vi "Calculate Total Tardiness for Brucker Instance.vi"() -> ()   [LabVIEW 2013]
uses:
  <vilib>/Heliosphere Research LLC/Advanced Plotting Toolkit/typedefs/PlotColor.ctl
  <vilib>/Heliosphere Research LLC/Advanced Plotting Toolkit/api_figure/TicksProperties.ctl
  <vilib>/Heliosphere Research LLC/Advanced Plotting Toolkit/properties/Text.ctl
  <vilib>/Heliosphere Research LLC/Advanced Plotting Toolkit/properties/Text_FontSize.ctl
  <vilib>/Heliosphere Research LLC/Advanced Plotting Toolkit/properties/Text_FontStyle.ctl
  <vilib>/Heliosphere Research LLC/Advanced Plotting Toolkit/api_annotations/ShapeProperties.ctl
  <vilib>/Heliosphere Research LLC/Advanced Plotting Toolkit/properties/Line.ctl
  <vilib>/Heliosphere Research LLC/Advanced Plotting Toolkit/properties/Line_Style.ctl
  <vilib>/Heliosphere Research LLC/Advanced Plotting Toolkit/properties/Display.ctl
  <vilib>/Heliosphere Research LLC/Advanced Plotting Toolkit/api_annotations/TextProperties.ctl
  Classes/Scheduler_Class/Check Other Machines for Schedule Time.vi
  Classes/Scheduler_Class/Schedule Job.vi
  Classes/Scheduler_Class/Find Gaps on Particular Machine.vi
  Classes/Scheduler_Class/Increment Number of Jobs on Machine.vi
  Classes/Scheduler_Class/Operation to Machine Job Tuple.vi
  Classes/Scheduler_Class/Find Job On Other Machines.vi
  Classes/Scheduler.lvclass
  <vilib>/Heliosphere Research LLC/Advanced Plotting Toolkit/Advanced Plotting Toolkit.lvlib
panel:
  out "Picture":picture
  out "sum":i32
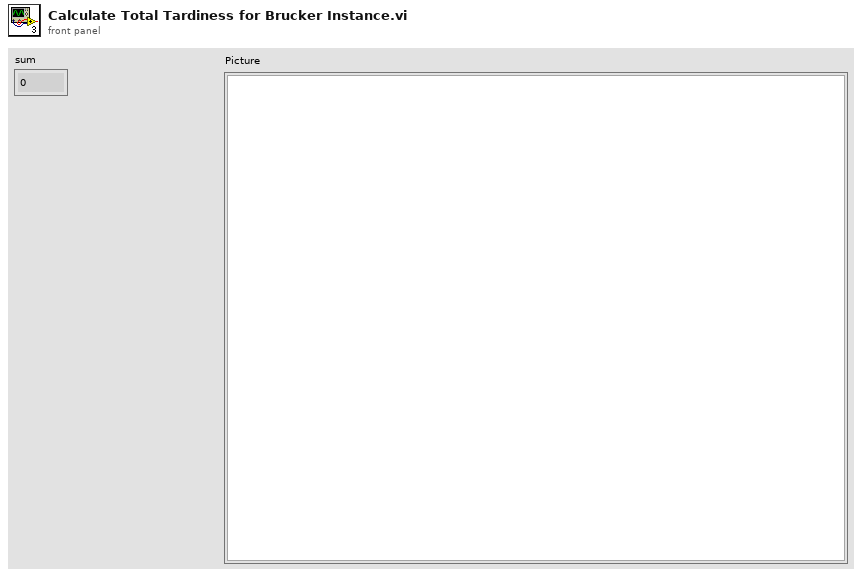
[diagram p1: front panel]
types:
  T1 = typedef "GanntChart_Element.ctl" = cluster{"Operation Number":i32, "Job Number":i32, "Start Time":i32, "Procesing Time":u16, "End Time":i32}
  T2 = typedef "Advanced Plotting Toolkit.lvlib/TicksProperties.ctl" = cluster{"Text":T3}
  T3 = typedef "Advanced Plotting Toolkit.lvlib/Text.ctl" = cluster{"Color":T4, "Background Color":T4, "Font Size (points)":T5, "Font Style":T6, "Rotation Angle":dbl}
  T4 = typedef "Advanced Plotting Toolkit.lvlib/PlotColor.ctl" = u32
  T5 = typedef "Advanced Plotting Toolkit.lvlib/Text_FontSize.ctl" = i32
  T6 = typedef "Advanced Plotting Toolkit.lvlib/Text_FontStyle.ctl" = enum16{"Automatic", "Normal", "Italic", "Bold"}
  T7 = typedef "Advanced Plotting Toolkit.lvlib/TextProperties.ctl" = cluster{"Text":T3, "Display":T8}
  T8 = typedef "Advanced Plotting Toolkit.lvlib/Display.ctl" = cluster{"Alpha":dbl, "Z Order":dbl}
  T9 = typedef "Advanced Plotting Toolkit.lvlib/ShapeProperties.ctl" = cluster{"Color":T4, "Line":T10, "Display":T8}
  T10 = typedef "Advanced Plotting Toolkit.lvlib/Line.ctl" = cluster{"Style":T11, "Color":T4, "Width":sgl}
  T11 = typedef "Advanced Plotting Toolkit.lvlib/Line_Style.ctl" = enum16{"Automatic", "Solid", "Dashed", "Dotted", "Dash-dot", "Invisible"}
  T12 = typedef "Advanced Plotting Toolkit.lvlib/PlotID.ctl" = i32
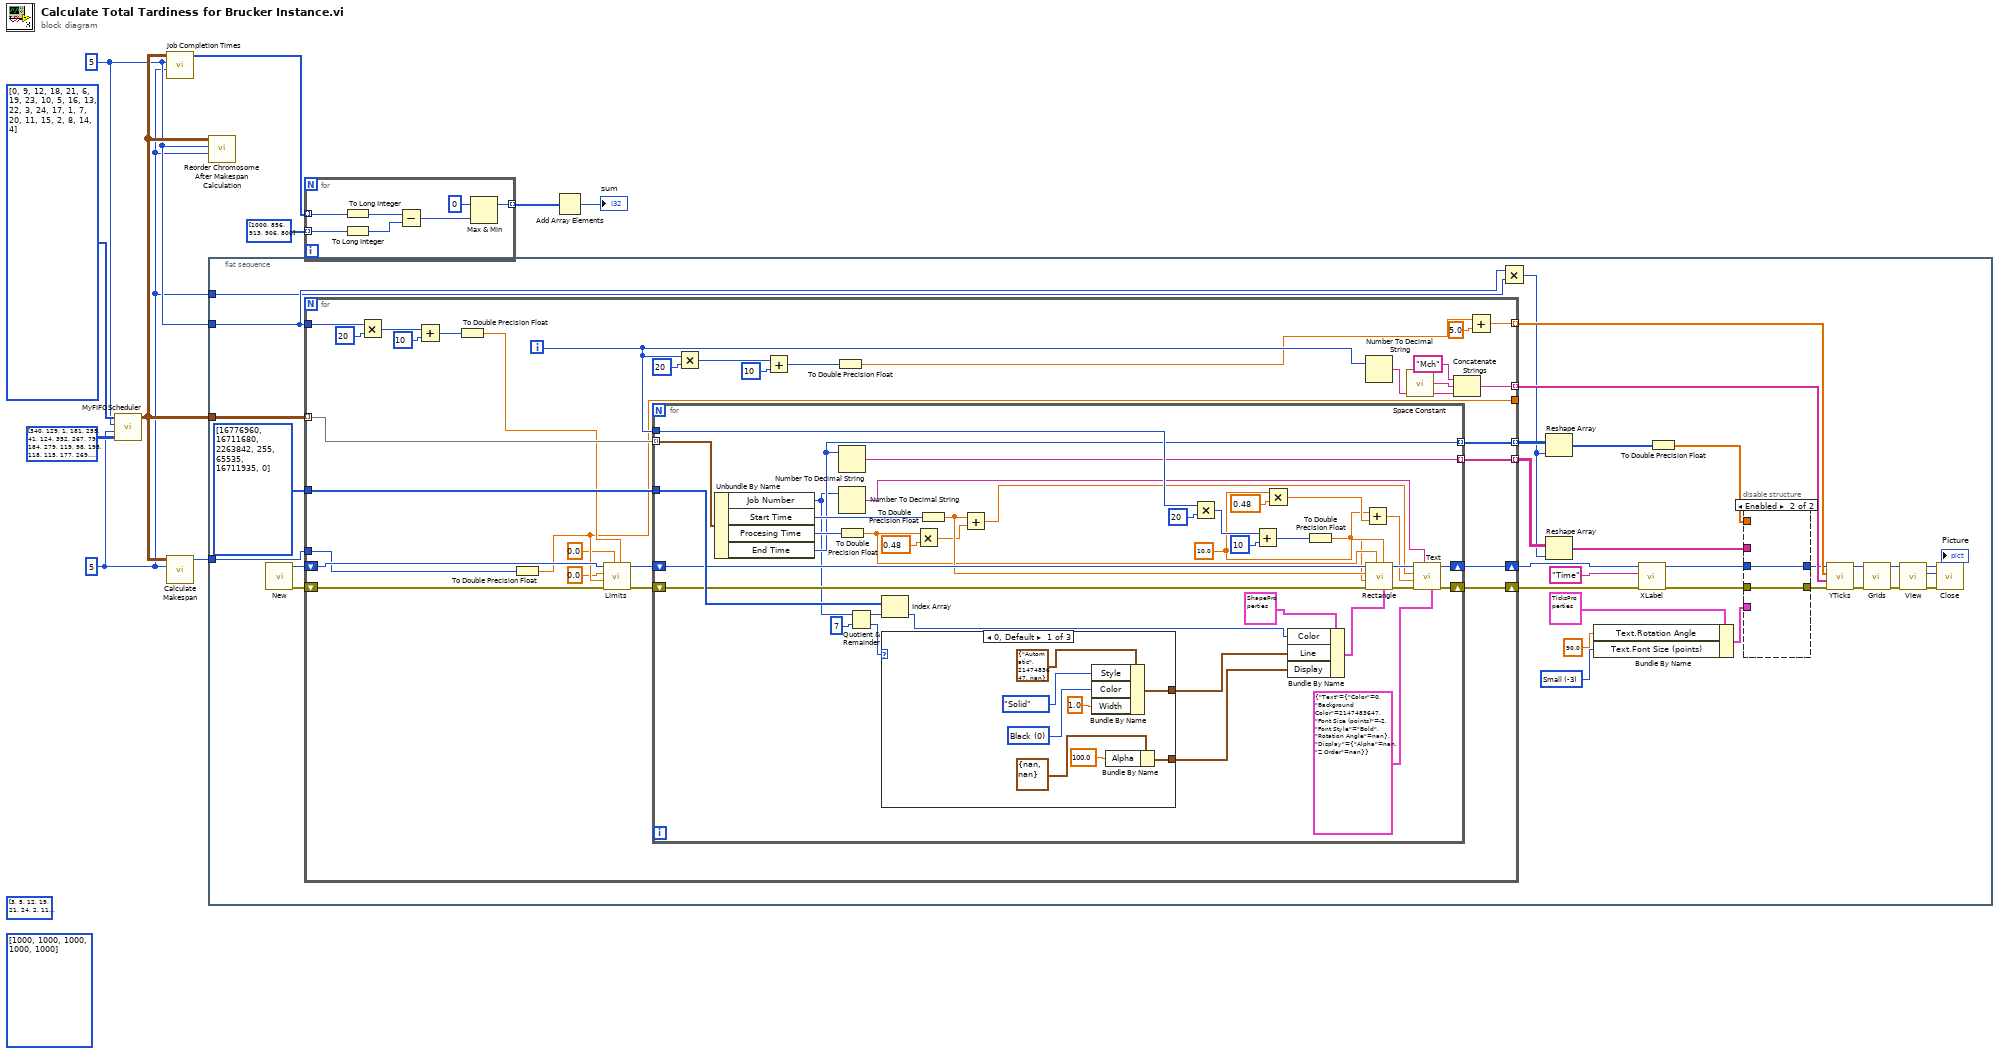
[diagram p0: block diagram]
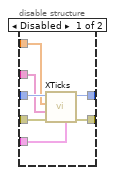
[diagram p2: hidden frame]
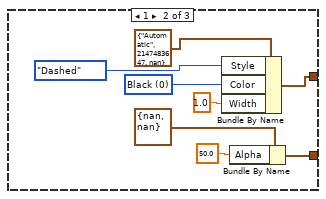
[diagram p3: hidden frame]
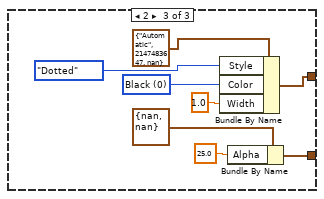
[diagram p4: hidden frame]
diagram:
  (unwired) u16[] [3, 5, 12, 19, 21, 24, 2, 11, 8, 15, 9, 23, 0, 17, 18, 22, 6, 14, 7, 1, 20, 16, 4, 13, 10] ("Schedule")
  (unwired) i32[] [1000, 1000, 1000, 1000, 1000]
  w1 = 5 ("Number of Jobs")
  w2 = 5 ("Number of Machines")
  n1 = call "MyFIFOScheduler.vi"("Processing Times (Rows Mach.Cols Jobs)"=u16[][] [[340, 129, 1, 181, 259], [41, 124, 352, 267, 79], [184, 279, 119, 98, 195], [118, 115, 177, 269, 148], [317, 209, 264, 91, 119]] ("Processing Times"), "Number of Jobs"=w1, "Number of Machines"=w2, "Schedule"=u16[] [0, 9, 12, 18, 21, 6, 19, 23, 10, 5, 16, 13, 22, 3, 24, 17, 1, 7, 20, 11, 15, 2, 8, 14, 4]) -> ("Gannt Chart Out"=w4:T1[][])  [unwired: 6 in, 1 out]
  n2 = call "Job Completion Times.vi"("Number Of Machines"=w1, "Number Of Jobs"=w2, "Gannt Chart In"=w4) -> ("Job Completion Times"=w8:u16[])  [unwired: 8 in]
  n3 = call "Calculate Makespan.vi"("Number of Jobs"=w1, "Gannt Chart In"=w4) -> ("Makespan"=w3:i32)  [unwired: 9 in]
  n4 = call "Reorder Chromosome  After Makespan Calculation.vi"("Number Of  Jobs"=w1, "Number Of Machines"=w2, "Gannt Chart In"=w4) -> ()  [unwired: 8 in, 1 out]
  n5 = flat-sequence {
    tunnel: w4 -> [w16]
    tunnel: w3 -> [w15]
    tunnel: w2 -> [w14]
    tunnel: w1 -> [w13]
    frame #0 {
      w20 = T5 -3 items=["Automatic"=0, "XX-Small"=-1, "X-Small"=-2, "Small"=-3, "Medium"=-4, "Large"=-5, "X-Large"=-6, "XX-Large"=-7] ("Text.Font Size (points)")
      w41 = T4[] [16776960, 16711680, 2263842, 255, 65535, 16711935, 0] items=["Automatic"=2147483647, "Black"=0, "White"=16777215, "Red"=16711680, "Green"=2263842, "Blue"=255, "Cyan"=65535, "Magenta"=16711935, "Yellow"=16776960]
      n6 = call <vilib>:"New.vi"() -> ("error out"=w42:errorcluster, "Plot ID"=w43:T12)  [unwired: 10 in]
      n7 = for {
        shift-right: [w84] -> w39
        shift-left: w42 -> [w80]
        shift-right: [w83] -> w40
        shift-left: w43 -> [w78]
        tunnel: w16 -> [w82] mode=indexing
        tunnel: w41 -> [w81]
        tunnel: [w70] -> w33 mode=indexing
        tunnel: [w60] -> w32 mode=indexing
        tunnel: [w59] -> w19 mode=indexing
        tunnel: [w58] -> w27 mode=indexing
        tunnel: [w57] -> _
        tunnel: w14 -> [w56]
        tunnel: w15 -> [w55]
        i -> [w63]
        n8 = Multiply(x=w56, y=20) -> (x*y=w76:i32)
        n9 = Add(x=w76, y=10) -> (x+y=w74:i32)
        n10 = To Double Precision Float(number=w74) -> (double precision float=w68:dbl)
        n11 = To Double Precision Float(number=w55) -> (double precision float=w57:dbl)
        n12 = call <vilib>:"Limits.vi"("Y Max"=w68, "Y Min"=0.0, "error in (no error)"=w80, "X Max"=w57, "X Min"=0.0, "Plot ID"=w78) -> ("error out"=w79:errorcluster, "Plot ID Out"=w73:T12)  [unwired: 4 in]
        n13 = for {
          shift-right: [w98] -> w84
          shift-left: w79 -> [w120]
          shift-right: [w100] -> w83
          shift-left: w73 -> [w119]
          tunnel: w82 -> [w122] mode=indexing
          tunnel: w81 -> [w121]
          tunnel: w63 -> [w109]
          tunnel: [w103] -> w59 mode=indexing
          tunnel: [w102] -> w58 mode=indexing
          w90 = 10.0 ("Height")
          n14 = Unbundle By Name(w122) -> ("Job Number"=w87:i32, "Start Time"=w114:i32, "Procesing Time"=w115:u16, "End Time"=w103:i32)
          n15 = Number To Decimal String(number=w103) -> (decimal integer string=w102:string)  [unwired: 1 in]
          n16 = Number To Decimal String(number=w87) -> (decimal integer string=w86:string)  [unwired: 1 in]
          n17 = To Double Precision Float(number=w115) -> (double precision float=w96:dbl)
          n18 = Quotient & Remainder(x=w87, y=7) -> (x-y*floor(x/y)=w106:i32, floor(x/y)=w105:i32)
          n19 = Index Array(array=w121, index=w106) -> (element=w116:T4)
          n20 = case shown="0, Default" w105 {
            tunnel: [w126 w134 w142] -> w108
            tunnel: [w123 w131 w139] -> w104
            frame 0, Default {
              w128 = T4 0 items=["Automatic"=2147483647, "Black"=0, "White"=16777215, "Red"=16711680, "Green"=2263842, "Blue"=255, "Cyan"=65535, "Magenta"=16711935, "Yellow"=16776960] ("Color")
              n21 = Bundle By Name(cluster=T10 {"Style"=enum."Automatic", "Color"=2147483647, "Width"=nan} ("Line"), "Style"=Line_Style."Solid", "Color"=w128, "Width"=sgl 1.0) -> (w126:T10)
              n22 = Bundle By Name(cluster=T8 {"Alpha"=nan, "Z Order"=nan} ("Display"), "Alpha"=100.0) -> (w123:T8)
            }
            frame 1 {
              w136 = T4 0 items=["Automatic"=2147483647, "Black"=0, "White"=16777215, "Red"=16711680, "Green"=2263842, "Blue"=255, "Cyan"=65535, "Magenta"=16711935, "Yellow"=16776960] ("Color")
              n23 = Bundle By Name(cluster=T10 {"Style"=enum."Automatic", "Color"=2147483647, "Width"=nan} ("Line"), "Style"=Line_Style."Dashed", "Color"=w136, "Width"=sgl 1.0) -> (w134:T10)
              n24 = Bundle By Name(cluster=T8 {"Alpha"=nan, "Z Order"=nan} ("Display"), "Alpha"=50.0) -> (w131:T8)
            }
            frame 2 {
              w144 = T4 0 items=["Automatic"=2147483647, "Black"=0, "White"=16777215, "Red"=16711680, "Green"=2263842, "Blue"=255, "Cyan"=65535, "Magenta"=16711935, "Yellow"=16776960] ("Color")
              n25 = Bundle By Name(cluster=T10 {"Style"=enum."Automatic", "Color"=2147483647, "Width"=nan} ("Line"), "Style"=Line_Style."Dotted", "Color"=w144, "Width"=sgl 1.0) -> (w142:T10)
              n26 = Bundle By Name(cluster=T8 {"Alpha"=nan, "Z Order"=nan} ("Display"), "Alpha"=25.0) -> (w139:T8)
            }
          }
          n27 = Multiply(x=w96, y=0.48) -> (x*y=w94:dbl)
          n28 = To Double Precision Float(number=w114) -> (double precision float=w97:dbl)
          n29 = Add(x=w97, y=w94) -> (x+y=w93:dbl)
          n30 = Multiply(x=w109, y=20) -> (x*y=w112:i32)
          n31 = Add(x=w112, y=10) -> (x+y=w110:i32)
          n32 = Multiply(x=w90, y=0.48) -> (x*y=w92:dbl)
          n33 = Bundle By Name(cluster=T9 {"Color"=2147483647, "Line"={"Style"=enum."Automatic", "Color"=2147483647, "Width"=nan}, "Display"={"Alpha"=nan, "Z Order"=nan}} ("Properties"), "Color"=w116, "Line"=w108, "Display"=w104) -> (w117:T9)
          n34 = To Double Precision Float(number=w110) -> (double precision float=w89:dbl)
          n35 = Add(x=w89, y=w92) -> (x+y=w88:dbl)
          n36 = call <vilib>:"Rectangle.vi"("Properties"=w117, "Height"=w90, "Width"=w96, "error in (no error)"=w120, "Y Position"=w89, "X Position"=w97, "Plot ID"=w119) -> ("error out"=w99:errorcluster, "Plot ID Out"=w101:T12)  [unwired: 3 in]
          n37 = call <vilib>:"Text.vi"("Properties"=T7 {"Text"={"Color"=0, "Background Color"=2147483647, "Font Size (points)"=-2, "Font Style"=enum."Bold", "Rotation Angle"=nan}, "Display"={"Alpha"=nan, "Z Order"=nan}}, "Text"=w86, "error in (no error)"=w99, "Y Position"=w88, "X Position"=w93, "Plot ID"=w101) -> ("error out"=w98:errorcluster, "Plot ID Out"=w100:T12)  [unwired: 4 in]
        }
        n38 = Multiply(x=w63, y=20) -> (x*y=w66:i32)
        n39 = Add(x=w66, y=10) -> (x+y=w64:i32)
        n40 = To Double Precision Float(number=w64) -> (double precision float=w62:dbl)
        n41 = Number To Decimal String(number=w63) -> (decimal integer string=w69:string)  [unwired: 1 in]
        n42 = call <vilib>:"Space Constant.vi"() -> ("String"=w71:string)
        n43 = Concatenate Strings("Mch", w71, w69) -> (w70:string)
        n44 = Add(x=w62, y=5.0) -> (x+y=w60:dbl)
      }
      n45 = Multiply(x=w14, y=w13) -> (x*y=w12:i32)
      n46 = Reshape Array(w19, w12) -> (w25:i32[])
      n47 = Reshape Array(w27, w12) -> (w26:string[])
      n48 = Bundle By Name(cluster=T2 {"Text"={"Color"=2147483647, "Background Color"=2147483647, "Font Size (points)"=0, "Font Style"=enum."Automatic", "Rotation Angle"=nan}} ("Properties"), "Text.Rotation Angle"=90.0, "Text.Font Size (points)"=w20) -> (w21:T2)
      n49 = call <vilib>:"XLabel.vi"("error in (no error)"=w39, "Label"="Time", "Plot ID"=w40) -> ("error out"=w29:errorcluster, "Plot ID out"=w31:T12)  [unwired: 7 in]
      n50 = To Double Precision Float(number=w25) -> (double precision float=w24:dbl[])
      n51 = disable-structure shown="Enabled" {
        disable-tunnel: w31 -> [w50 w52]
        disable-tunnel: [w49 w52] -> w30
        disable-tunnel: w29 -> [w48 w51]
        disable-tunnel: [w47 w51] -> w28
        disable-tunnel: w26 -> [w46 _]
        disable-tunnel: w24 -> [w45 _]
        disable-tunnel: w21 -> [w44 _]
        frame Disabled {
          n52 = call <vilib>:"XTicks.vi"("Properties"=w44, "error in (no error)"=w48, "Tick Labels"=w46, "Tick Locations"=w45, "Plot ID"=w50) -> ("error out"=w47:errorcluster, "Plot ID Out"=w49:T12)  [unwired: 5 in]
        }
        frame Enabled {
        }
      }
      n53 = call <vilib>:"YTicks.vi"("error in (no error)"=w28, "Tick Labels"=w33, "Tick Locations"=w32, "Plot ID"=w30) -> ("error out"=w35:errorcluster, "Plot ID Out"=w34:T12)  [unwired: 6 in]
      n54 = call <vilib>:"Grids.vi"("error in (no error)"=w35, "Plot ID"=w34) -> ("error out"=w38:errorcluster, "Plot ID Out"=w36:T12)  [unwired: 8 in]
      n55 = call <vilib>:"View.vi"("error in (no error)"=w38, "Plot ID"=w36) -> ("error out"=w17:errorcluster, "Picture"=→"Picture":picture, "Plot ID Out"=w18:T12)  [unwired: 7 in]
      n56 = call <vilib>:"Close.vi"("error in (no error)"=w17, "Plot ID"=w18) -> ()  [unwired: 9 in, 1 out]
    }
  }
  n57 = for {
    tunnel: [w151] -> w9 mode=indexing
    tunnel: w8 -> [w148] mode=indexing
    tunnel: u16[] [1000, 856, 913, 906, 800] ("Due Dates") -> [w147] mode=indexing
    n58 = To Long Integer(number=w148) -> (32bit integer=w149:i32)
    n59 = To Long Integer(number=w147) -> (32bit integer=w150:i32)
    n60 = Subtract(x=w149, y=w150) -> (x-y=w153:i32)
    n61 = Max & Min(x=0, y=w153) -> (max(x,y)=w151:i32)  [unwired: 1 out]
  }
  n62 = Add Array Elements(numeric array=w9) -> (sum=→"sum":i32)
